vi "Find All Device of Type X Ports Paths.vi"(0 "Unique Notifier Names":string[](array[string]), 5 "Device Port/ID/Channel Info":string[][](array[string]), 7 "Device Engine Paths":path[](array[path]), 11 "Device Type":T1=enum."Stage") -> (8 "Running Devices":string[](array[string]), 10 "All Ports":string[][](array[string]), 13 "All Devices":string[](array[string]), 15 "All Paths":path[](array[path]))   [LabVIEW 2020]
uses:
  Hardware Configuration Controls/Device Type.ctl
  <vilib>/regexp/Match Regular Expression.xnode
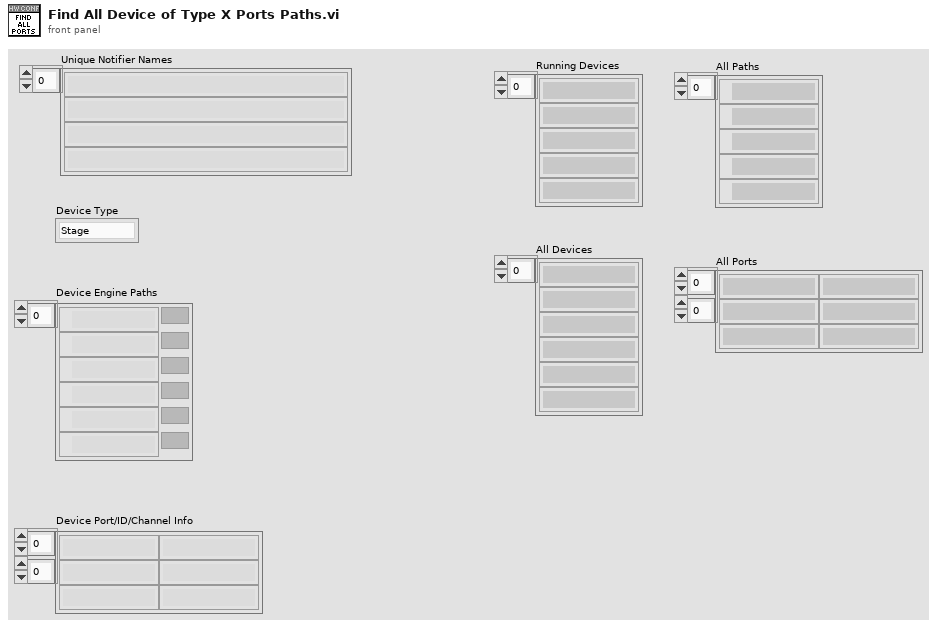
[diagram p1: front panel]
types:
  T1 = typedef "Device Type.ctl" = enum16{"AOTF", "Camera", "Deformable Mirror", "Laser", "Microscope Base", "Shutter", "Stage", "Waveform", "FPGA", "Email", "Filter Wheel", "Spinning Disk"}
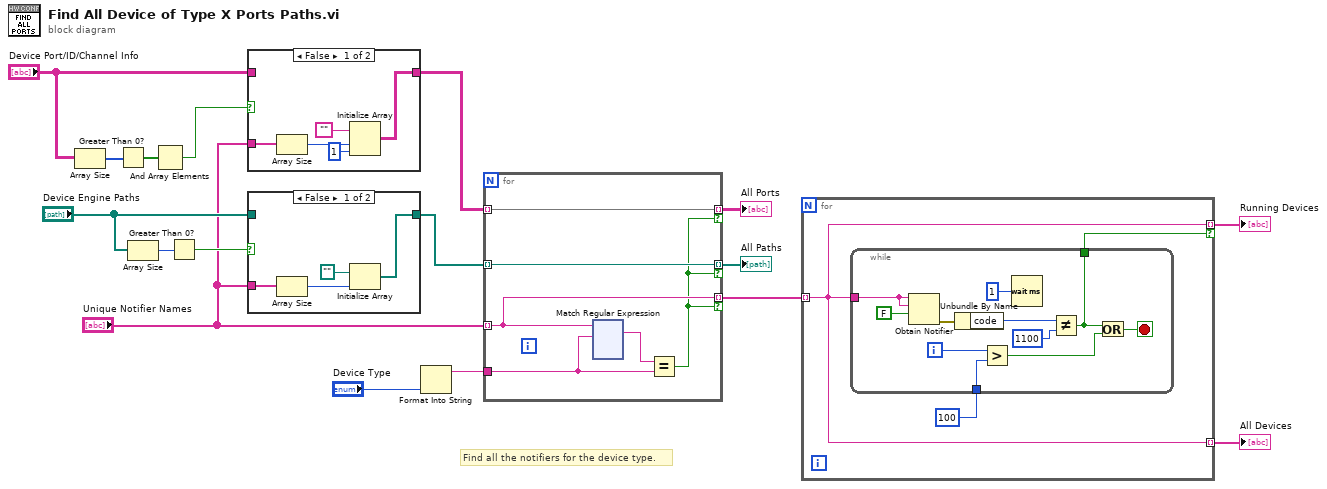
[diagram p0: block diagram]
diagram:
  # "Find all the notifiers for the device type."
  n1 = Array Size(array="Device Port/ID/Channel Info") -> (size(s)=w5:i32[])
  n2 = Greater Than 0?(x=w5) -> (x > 0?=w4:bool[])
  n3 = Array Size(array="Device Engine Paths") -> (size(s)=w11:i32)
  n4 = And Array Elements(Boolean array=w4) -> (logical AND=w3:bool)
  n5 = Greater Than 0?(x=w11) -> (x > 0?=w10:bool)
  n6 = case shown="False" w3 {
    tunnel: "Device Port/ID/Channel Info" -> [_ w23]
    tunnel: [w20 w23] -> w2
    tunnel: "Unique Notifier Names" -> [w22 _]
    frame False {
      n7 = Array Size(array=w22) -> (size(s)=w21:i32)
      n8 = Initialize Array("", w21, 1 ("dimension size")) -> (w20:string[][])
    }
    frame True {
    }
  }
  n9 = case shown="False" w10 {
    tunnel: "Device Engine Paths" -> [_ w28]
    tunnel: [w24 w28] -> w8
    tunnel: "Unique Notifier Names" -> [w27 _]
    frame False {
      n10 = Array Size(array=w27) -> (size(s)=w26:i32)
      n11 = Initialize Array(path "", w26) -> (w24:path[])
    }
    frame True {
    }
  }
  n12 = Format Into String("Device Type") -> (resulting string=w16:string)  [unwired: 3 in, 1 out]
  n13 = for {
    tunnel: "Unique Notifier Names" -> [w33] mode=indexing
    tunnel: [w33] -> w15 mode=indexing if=w29
    tunnel: w16 -> [w32]
    tunnel: w8 -> [w31] mode=indexing
    tunnel: [w31] -> w12 mode=indexing if=w29
    tunnel: w2 -> [w30] mode=indexing
    tunnel: [w30] -> w1 mode=indexing if=w29
    n14 = xnode "Match Regular Expression"("input string"=w33, "regular expression"=w32) -> ("whole match"=w34:string)  [unwired: 4 in, 4 out]
    n15 = Equal?(x=w34, y=w32) -> (x = y?=w29:bool)
  }
  "All Paths" <- w12
  "All Ports" <- w1
  n16 = for {
    tunnel: w15 -> [w150] mode=indexing
    tunnel: [w150] -> w14 mode=indexing if=w149
    tunnel: [w150] -> w13 mode=indexing
    n17 = while {
      tunnel: [w154] -> w149
      tunnel: 100 ("Wait Time (ms)") -> [w153]
      tunnel: w150 -> [w152]
      i -> [w160]
      stop <- w155 stop-if-true
      n18 = Obtain Notifier(name (unnamed)=w152, notification data type=w152, create if not found? (T)=FALSE) -> (error out=w161:errorcluster)  [unwired: 1 in, 2 out]
      n19 = Unbundle By Name(w161) -> ("code"=w159:i32)
      n20 = Greater?(x=w160, y=w153) -> (0:w156:bool)
      n21 = Wait (ms)(milliseconds to wait=u32 1) -> ()  [unwired: 1 out]
      n22 = Not Equal?(x=w159, y=1100) -> (x != y?=w154:bool)
      n23 = Or(x=w154, y=w156) -> (x .or. y?=w155:bool)
    }
  }
  "Running Devices" <- w14
  "All Devices" <- w13
